vi "DAQ_Dig PWM Meas Configure and Measure.vi"(0 "DAQmx Task In":refnum<k21>, 2 "Execution Option":T1, 5 "Cycles to capture":i32=2 min=2 step=1, 11 "error in":errorcluster) -> (4 "DAQmx Task Out":refnum<k21>, 6 "Digital PWM Measurements":T2 {"Frequency (Hz)" format="%.6p"; "Duty Cycle (%)" min=0.0 max=100.0 format="%#.2p"; "Low Time (s)" format="%.2p"; "High Time (s)" format="%.2p"}, 8 "Actual Cycles Captured":i32, 15 "error out":errorcluster)   [LabVIEW 2021, in "DAQ_Digital PWM Measurement.lvlib"]
doc: "Configure, initiate, and fetch digital PWM measurements from the channels configured.\n\n<B>Note:</B> The default timeout for PWM Measurements is 10 seconds. If the time elapses before the requested cycles are captured, the VI returns a error. Users can manually edit this timeout based on the captured PWM signal time period."
uses:
  DAQ_Digital PWM Measurement.lvlib
  Typedefs/Digital PWM Measurements.ctl
  Common/Typedefs/Execution Options - Measure.ctl
  <vilib>/DAQmx/read.llb/DAQmx Read (Counter 1D DBL 1Chan NSamp).vi
  <vilib>/DAQmx/configure/timing.llb/DAQmx Timing (Implicit).vi
  <vilib>/DAQmx/miscellaneous.llb/DAQmx Fill In Error Info.vi
  <resource>/objmgr/daqmx.rc
panel:
  # "Outputs"
  # "Inputs"
  # "Measurement Settings"
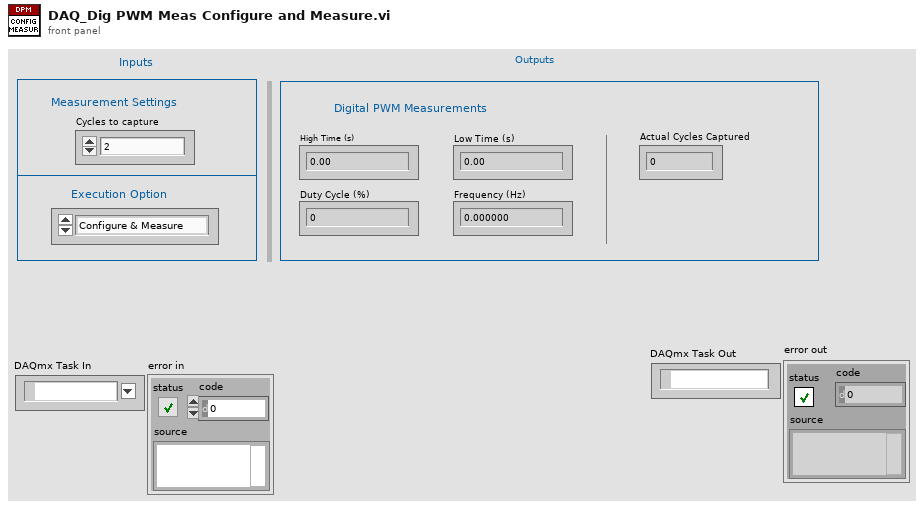
[diagram p1: front panel]
types:
  T1 = typedef "Execution Options - Measure.ctl" = enum16{"Configure & Measure", "Configure only", "Measure only"}
  T2 = typedef "DAQ_Digital PWM Measurement.lvlib/Digital PWM Measurements.ctl" = cluster{"High Time (s)":dbl, "Low Time (s)":dbl, "Duty Cycle (%)":dbl, "Frequency (Hz)":dbl}
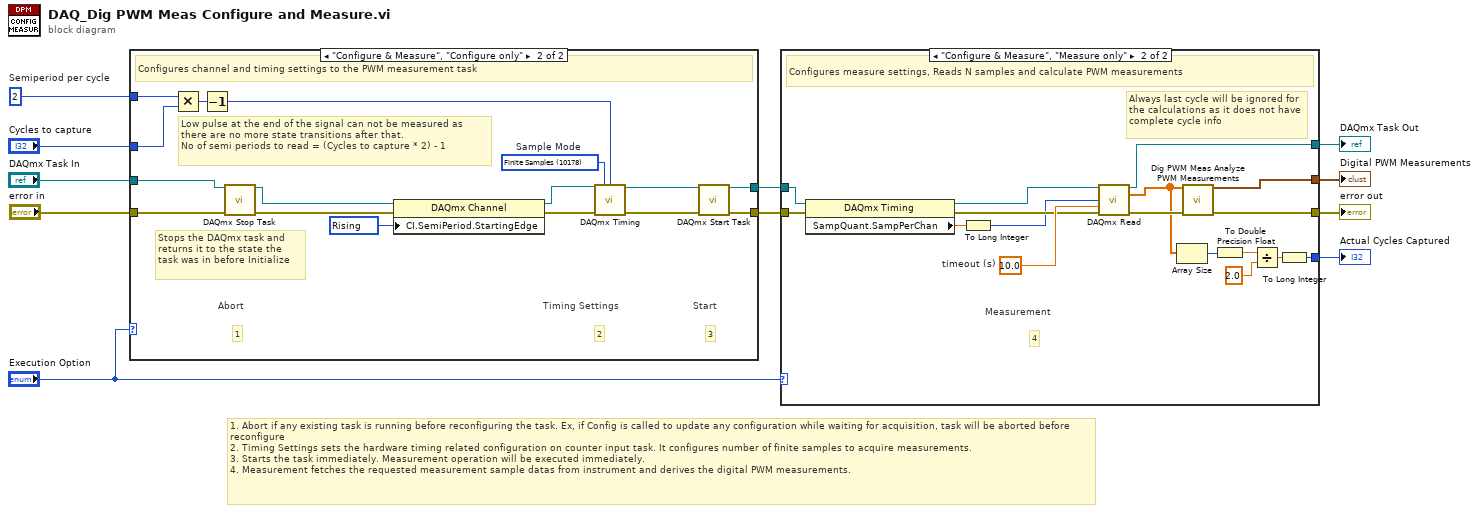
[diagram p0: block diagram]
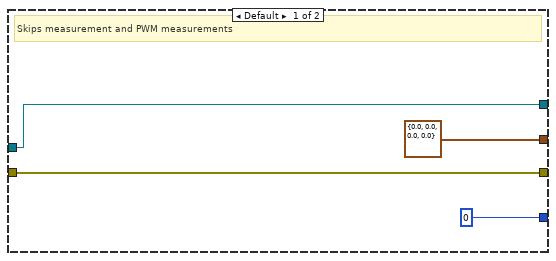
[diagram p3: hidden frame]
diagram:
  w4 = 2  # Semiperiod per cycle
  # "1. Abort if any existing task is running before reconfiguring the task. Ex, if Config is called to update any configuration while waiting for acquisition, task will be aborted before reconfigure\n2. Timing Settings sets the hardware timing related configuration on counter input task. It configures number of finite samples to acquire measurements.\n3. Starts the task immediately. Measurement operation will be executed immediately.\n4. Measurement fetches the requested measurement sample datas from instrument and derives the digital PWM measurements."
  n1 = case shown="\"Configure & Measure\", \"Configure only\"" "Execution Option" {
    tunnel: "DAQmx Task In" -> [w13 w29]
    tunnel: "error in" -> [w12 w28]
    tunnel: [w13 w25] -> w9
    tunnel: [w12 w24] -> w8
    tunnel: w4 -> [_ w17]
    tunnel: "Cycles to capture" -> [_ w15]
    frame Default {
      # "Skips configurations"
    }
    frame "Configure & Measure", "Configure only" {
      w18 = 10280 items=["Rising"=10280, "Falling"=10171] ("CI.SemiPeriod.StartingEdge")
      w26 = 10178 items=["Finite Samples"=10178, "Continuous Samples"=10123, "Hardware Timed Single Point"=12522]  # Sample Mode
      # "Low pulse at the end of the signal can not be measured as there are no more state transitions after that.\nNo of semi periods to read = (Cycles to capture * 2) - 1"
      # "Stops the DAQmx task and returns it to the state the task was in before Initialize"
      # "3"
      # "Start"
      # "1"
      # "Abort"
      # "2"
      # "Timing Settings"
      # "Configures channel and timing settings to the PWM measurement task"
      n2 = Multiply(x=w17, y=w15) -> (x*y=w16:i32)
      n3 = Decrement(x=w16) -> (x-1=w14:i32)
      n4 = call <vilib>:"DAQmx Stop Task.vi"("task/channels in"=w29, "error in"=w28) -> ("task out"=w21:refnum<k21>, "error out"=w27:errorcluster)  [unwired: 12 in]
      n5 = property class="DAQmx Channel"(reference=w21, error in=w27, "CI.SemiPeriod.StartingEdge"=w18) -> (reference out=w19:refnum<k21>, error out=w20:errorcluster)
      n6 = call-poly <vilib>:"DAQmx Timing.vi"("task/channels in"=w19, "sample mode"=w26, "samples per channel"=w14, "error in"=w20) -> ("task out"=w23:refnum<k21>, "error out"=w22:errorcluster)  [unwired: 10 in]
      n7 = call <vilib>:"DAQmx Start Task.vi"("task/channels in"=w23, "error in"=w22) -> ("task out"=w25:refnum<k21>, "error out"=w24:errorcluster)  [unwired: 12 in]
    }
  }
  n8 = case shown="\"Configure & Measure\", \"Measure only\"" "Execution Option" {
    tunnel: w9 -> [w32 w43]
    tunnel: w8 -> [w33 w50]
    tunnel: [T2 {"High Time (s)"=0.0, "Low Time (s)"=0.0, "Duty Cycle (%)"=0.0, "Frequency (Hz)"=0.0} ("Digital PWM Measurements") w49] -> w7
    tunnel: [w33 w47] -> w6
    tunnel: [w32 w46] -> w5
    tunnel: [0 w38] -> w1
    frame Default {
      # "Skips measurement and PWM measurements"
    }
    frame "Configure & Measure", "Measure only" {
      w45 = 10.0  # timeout (s)
      # "Always last cycle will be ignored for the calculations as it does not have complete cycle info"
      # "4"
      # "Measurement"
      # "Configures measure settings, Reads N samples and calculate PWM measurements"
      n9 = property class="DAQmx Timing"(reference=w43, error in=w50) -> (reference out=w42:refnum<k21>, error out=w44:errorcluster, "SampQuant.SampPerChan"=w36:dbl)
      n10 = To Long Integer(number=w36) -> (32bit integer=w34:i32)
      n11 = call-poly <vilib>:"DAQmx Read.vi"("task/channels in"=w42, "number of samples per channel"=w34, "timeout"=w45, "error in"=w44) -> ("task out"=w46:refnum<k21>, "data"=w41:dbl[], "error out"=w48:errorcluster)  [unwired: 9 in]
      n12 = Array Size(array=w41) -> (size(s)=w40:i32)
      n13 = call "Dig PWM Meas Analyze PWM Measurements.vi"("Semiperiod Measurements (s)"=w41, "error in (no error)"=w48) -> ("Digital PWM Measurements"=w49:T2, "error out"=w47:errorcluster)  [unwired: 12 in]
      n14 = To Double Precision Float(number=w40) -> (double precision float=w37:dbl)
      n15 = Divide(x=w37, y=2.0) -> (x/y=w39:dbl)
      n16 = To Long Integer(number=w39) -> (32bit integer=w38:i32)
    }
  }
  "error out" <- w6
  "DAQmx Task Out" <- w5
  "Digital PWM Measurements" <- w7
  "Actual Cycles Captured" <- w1
